vi "调用WinProladder.vi"(8 "错误输入（无错误）":errorcluster) -> (0 "错误输出":errorcluster)   [LabVIEW 2016, in "PLC.lvlib"]
uses:
  PLC.lvlib
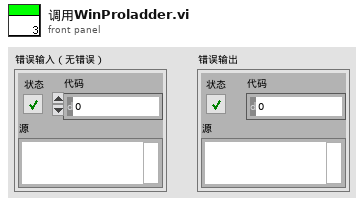
[diagram p1: front panel]
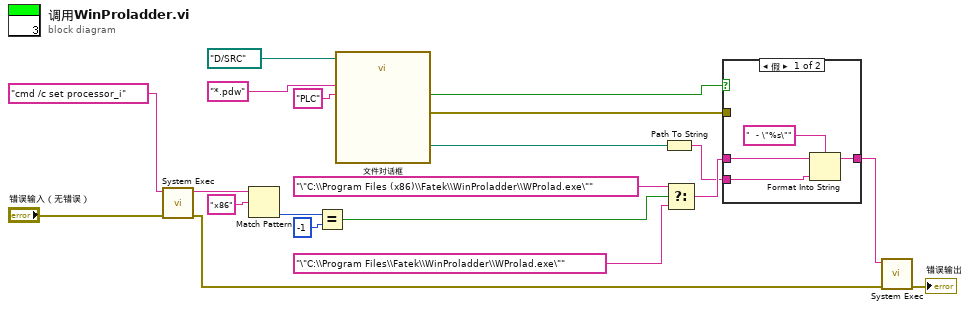
[diagram p0: block diagram]
diagram:
  n1 = call <vilib>:"System Exec.vi"("error in (no error)"="错误输入（无错误）", "command line"="cmd /c set processor_i") -> ("error out"=w17:errorcluster, "standard output"=w9:string)  [unwired: 6 in, 2 out]
  n2 = Match Pattern(string=w9, regular expression="x86" ("正则表达式")) -> (offset past match=w11:i32)  [unwired: 1 in, 3 out]
  n3 = Equal?(x=w11, y=-1) -> (x = y?=w13:bool)
  n4 = call "文件对话框"("start path"=path "D:/SRC", "pattern (all files)"="*.pdw", "pattern label"="PLC") -> ("selected path"=w2:path, "cancelled"=w20:bool, "error out"=w1:errorcluster)  [unwired: 9 in, 1 out]
  n5 = Path To String(path=w2) -> (string=w7:string)
  n6 = Select(t="\"C:\\Program Files (x86)\\Fatek\\WinProladder\\WProlad.exe\"" ("command line"), s=w13, f="\"C:\\Program Files\\Fatek\\WinProladder\\WProlad.exe\"" ("command line")) -> (s? t:f=w16:string)
  n7 = case shown="假" w20 {
    tunnel: [w23 w25] -> w6
    tunnel: w7 -> [w22 _]
    tunnel: w16 -> [w21 w25]
    tunnel: w1 -> [_ _]
    frame False {
      n8 = Format Into String(format string="  - \"%s\"" ("格式字符串"), initial string=w21, w22) -> (resulting string=w23:string)  [unwired: 1 in, 1 out]
    }
    frame True {
    }
  }
  n9 = call <vilib>:"System Exec.vi"("error in (no error)"=w17, "command line"=w6) -> ("error out"=→"错误输出":errorcluster)  [unwired: 6 in, 3 out]
